vi "getGlyphFile.vi"(8 "error in (no error)":errorcluster, 11 "FPGADMAChannelData in":refnum<class "FPGADMAChannelData.lvclass">) -> (0 "error out":errorcluster, 2 "Glyph File":string, 3 "FPGADMAChannelData out":refnum<class "FPGADMAChannelData.lvclass">)   [LabVIEW 2013, in "FPGADMAChannelData.lvclass"]
doc: "Dynamic Dispatch VI. Returns the name of the glyph file to be used as a glyph in the tree control. A empty string means no glyph."
uses:
  FPGADMAChannelData.lvclass
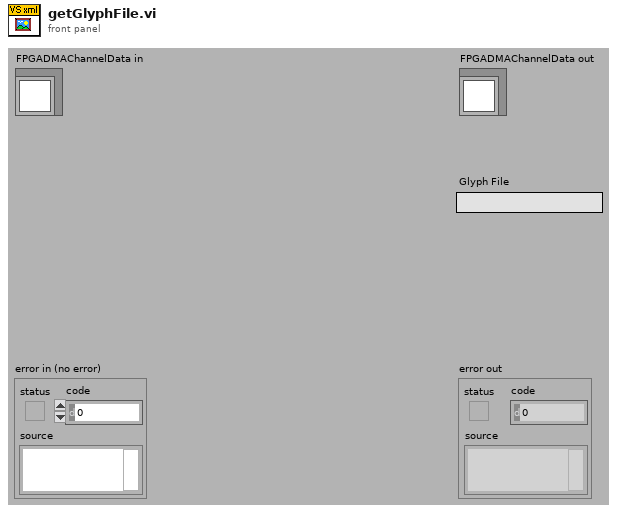
[diagram p1: front panel]
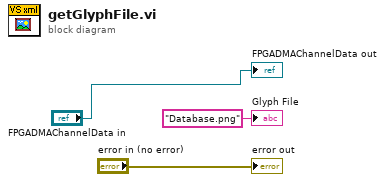
[diagram p0: block diagram]
diagram:
  "error out" <- "error in (no error)"
  "FPGADMAChannelData out" <- "FPGADMAChannelData in"
  "Glyph File" <- "Database.png" ("Glyph File")
